vi "Counter.vi"(8 "error constant":errorcluster, 11 "Count/Reset":bool) -> (0 "error constant 2":errorcluster, 3 "Count":dbl)   [LabVIEW 2022 SP3]
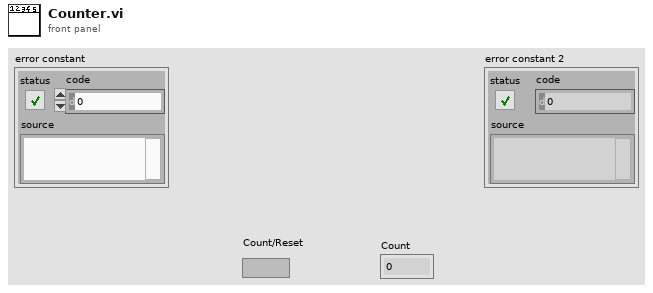
[diagram p1: front panel]
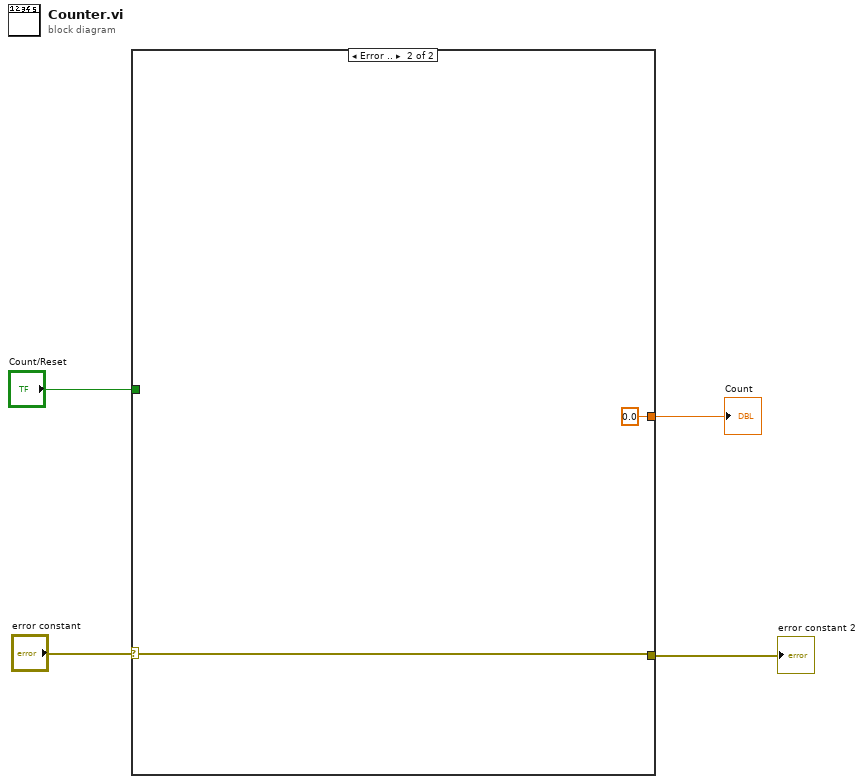
[diagram p0: block diagram]
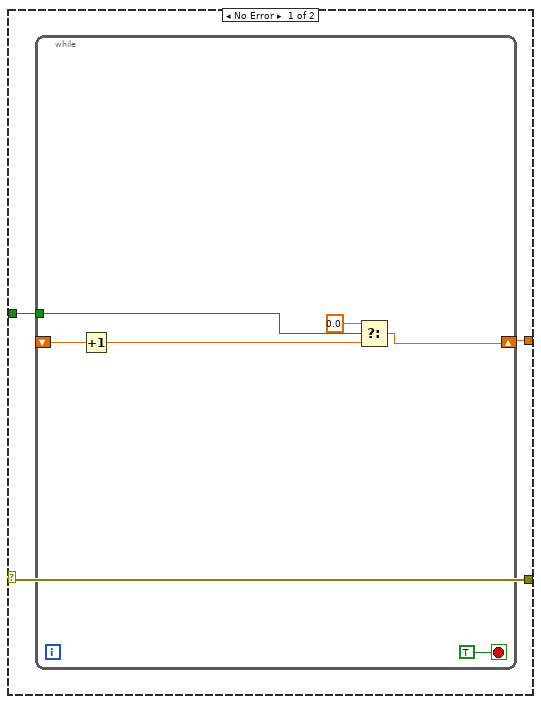
[diagram p2: hidden frame]
diagram:
  n1 = case shown="Error .." "error constant" {
    selector: "error constant" -> [w7 w15]
    tunnel: [w7 w15] -> w3
    tunnel: [w6 0.0 ("t")] -> w2
    tunnel: "Count/Reset" -> [w5 _]
    frame No Error {
      n2 = while {
        shift-right: [w10] -> w6
        shift-left: _ -> [w12]
        tunnel: w5 -> [w9]
        stop <- TRUE stop-if-true
        n3 = Increment(x=w12) -> (x+1=w11:dbl)
        n4 = Select(t=0.0, s=w9, f=w11) -> (s? t:f=w10:dbl)
      }
    }
    frame Error {
    }
  }
  "Count" <- w2
  "error constant 2" <- w3
